vi "dvp Vi Get Trigger Input Type.vi"(10 "pTriggerInputType":u32(ring) items=["TRIGGER_IN_OFF", "TRIGGER_NEG_EDGE", "TRIGGER_LOW_LEVEL", "TRIGGER_POS_EDGE", "TRIGGER_HIGH_LEVEL"], 11 "handle":u32) -> (2 "pTriggerInputType out":u32(ring) items=["TRIGGER_IN_OFF", "TRIGGER_NEG_EDGE", "TRIGGER_LOW_LEVEL", "TRIGGER_POS_EDGE", "TRIGGER_HIGH_LEVEL"], 3 "function return":u32(ring))   [LabVIEW 2018, in "LabViewDVPCamera.lvlib"]
doc: "LabviewDvp2Api dvpStatus dvpViGetTriggerInputType(dvpHandle handle, dvpTriggerInputType *pTriggerInputType);"
uses:
  LabViewDVPCamera.lvlib
  LabViewDVPCamera/LabViewDVPCamera.dll
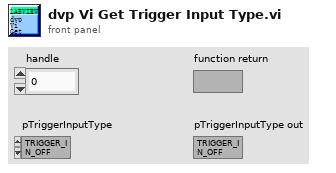
[diagram p1: front panel]
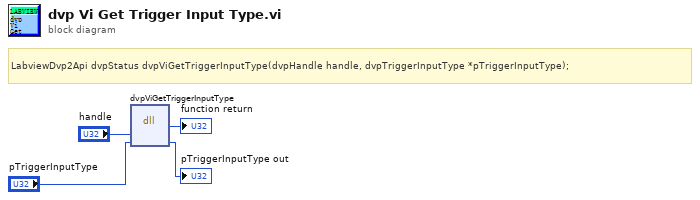
[diagram p0: block diagram]
diagram:
  # "LabviewDvp2Api dvpStatus dvpViGetTriggerInputType(dvpHandle handle, dvpTriggerInputType *pTriggerInputType);"
  n1 = dll-call lib="C:/Program Files (x86)/DVP2 Labview cn 64/Sample/LabViewDVPCamera/LabViewDVPCamera.*" fn="dvpViGetTriggerInputType"("handle"="handle", "pTriggerInputType"="pTriggerInputType") -> (→"function return":u32, "pTriggerInputType"=→"pTriggerInputType out":u32)  [unwired: 4 in, 2 out]
